vi "Read Time.vi"(8 "error in (no error)":errorcluster, 11 "MenuSelectionMsg in":refnum<class "MenuSelectionMsg.lvclass">) -> (0 "error out":errorcluster, 2 "Time":u32, 3 "MenuSelectionMsg out":refnum<class "MenuSelectionMsg.lvclass">)   [LabVIEW 2018, in "MVA Framework.lvlib" / "ActorEvents.lvlib" / "MenuSelectionMsg.lvclass"]
uses:
  MenuSelectionMsg.lvclass
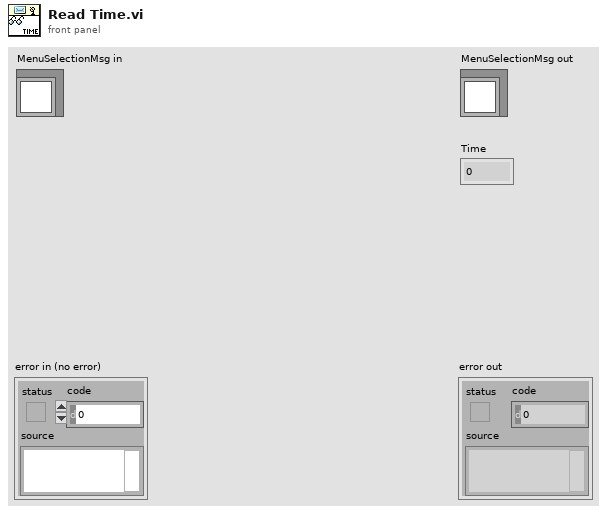
[diagram p1: front panel]
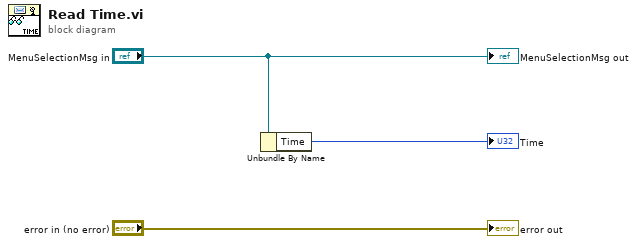
[diagram p0: block diagram]
diagram:
  n1 = Unbundle By Name("MenuSelectionMsg in") -> ("Time"=→"Time":u32)
  "error out" <- "error in (no error)"
  "MenuSelectionMsg out" <- "MenuSelectionMsg in"
